vi "circularCounter.vi"(7 "reset":bool, 9 "doStep":bool=TRUE, 11 "maxCount":u16) -> (0 "maxReached":bool, 1 "maxPulse":bool, 2 "next":u16, 3 "index":u16)   [LabVIEW 2016]
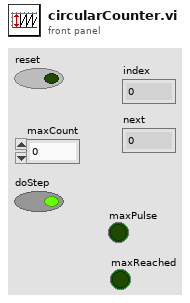
[diagram p1: front panel]
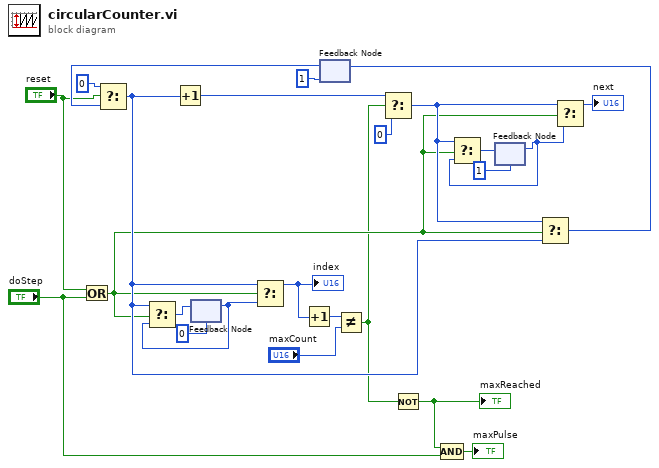
[diagram p0: block diagram]
diagram:
  n1 = Or(x="reset", y="doStep") -> (x .or. y?=w5:bool)
  n2 = feedback #1(u16 0 ("t")) -> (w15:u16)
  n3 = feedback #2(u16 1) -> (w22:u16)
  n4 = Select(t=u16 0, s="reset", f=w22) -> (s? t:f=w16:u16)
  n5 = Select(t=w16, s=w5, f=w15) -> (s? t:f=w17:u16)
  n6 = Increment(x=w16) -> (x+1=w23:u16)
  n7 = feedback-in #1(w17) -> ()
  n8 = Select(t=w16, s=w5, f=w15) -> (s? t:f=w4:u16)
  "index" <- w4
  n9 = Increment(x=w4) -> (x+1=w3:u16)
  n10 = Not Equal?(x=w3, y="maxCount") -> (x != y?=w1:bool)
  n11 = Select(t=w23, s=w1, f=u16 0) -> (s? t:f=w14:u16)
  n12 = Not(x=w1) -> (.not. x?=w8:bool)
  "maxReached" <- w8
  n13 = Compound Arithmetic op=AND(w8, "doStep") -> (→"maxPulse":bool)
  n14 = feedback #3(u16 1) -> (w12:u16)
  n15 = Select(t=w14, s=w5, f=w12) -> (s? t:f=w13:u16)
  n16 = feedback-in #3(w13) -> ()
  n17 = Select(t=w14, s=w5, f=w16) -> (s? t:f=w20:u16)
  n18 = feedback-in #2(w20) -> ()
  n19 = Select(t=w14, s=w5, f=w12) -> (s? t:f=→"next":u16)
